vi "Default Text Formats.vi"(8 "Error In":errorcluster, 11 "Theme (Light)":string="Light Theme") -> (0 "Error Out":errorcluster, 1 "Base Themes":T1[](array[typedef]) {"[Named Text Styles]"."Text Formatting"."Font Size" min=6.0 step=1.0}, 3 "Notebook Theme":T1 {"[Named Text Styles]"."Text Formatting"."Font Size" min=6.0 step=1.0})   [LabVIEW 2021, in "Notebook.lvlib"]
uses:
  Notebook.lvlib
  Notebook Theme.ctl
  Rich Text Box/Named Text Style.ctl
  Rich Text Box/Text Formatting.ctl
  Rich Text Box/Text Colors.ctl
  Rich Text Box/Text Style.ctl
  Rich Text Box/Text Alignment.ctl
  Rich Text Box/Rich Text Box.lvlib
panel:
  # "see the License on the block diagram (Ctrl+E or Window:Show Block Diagram)"
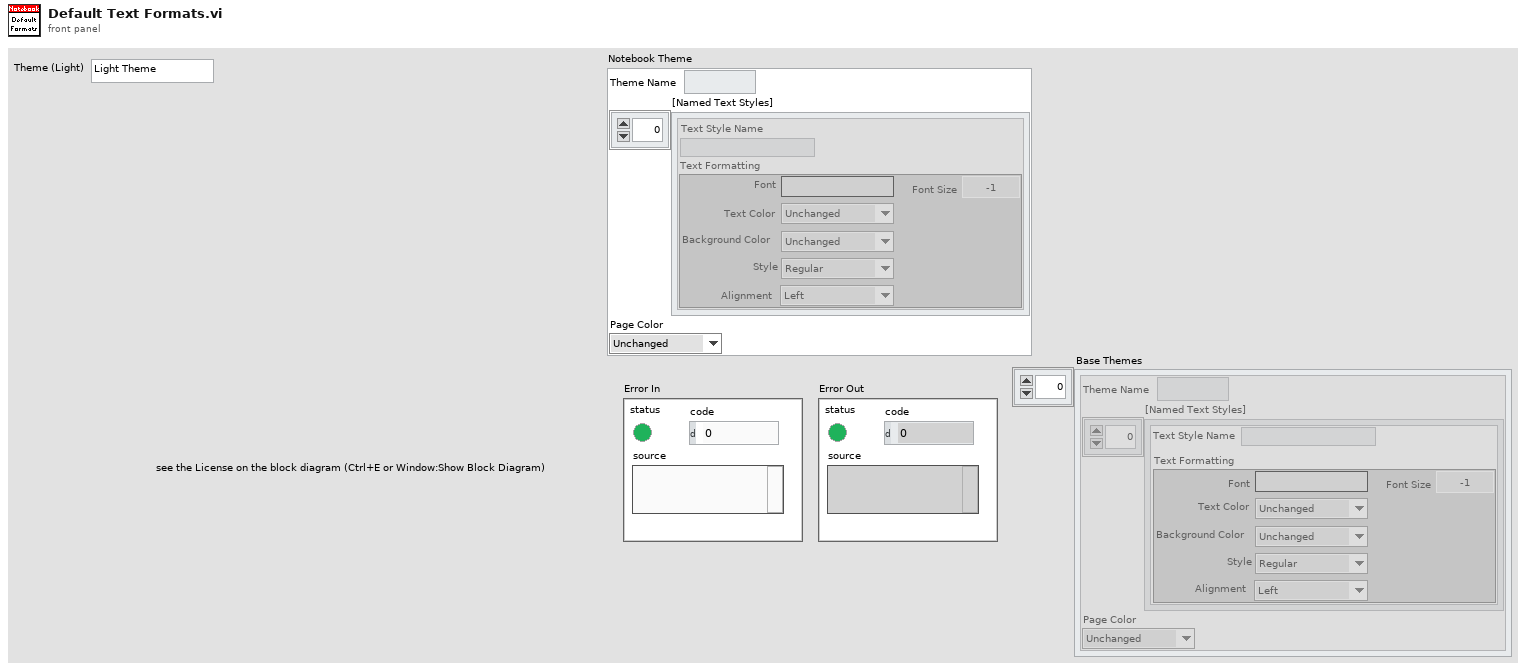
[diagram p1: front panel]
types:
  T1 = typedef "Notebook.lvlib/Notebook Theme.ctl" = cluster{"Theme Name":string, "[Named Text Styles]":T2[], "Page Color":T4}
  T2 = typedef "Notebook.lvlib/Named Text Style.ctl" = cluster{"Text Formatting":T3, "Text Style Name":string}
  T3 = typedef "Rich Text Box.lvlib/Text Formatting.ctl" = cluster{"Font":string, "Text Color":T4, "Background Color":T4, "Style":T5, "Font Size":dbl, "Alignment":T6}
  T4 = typedef "Rich Text Box.lvlib/Text Colors.ctl" = enum16{"Unchanged", "Black", "Blue", "Cyan", "Maroon", "Gray", "Violet", "Green", "Light Green", "Orange", "Yellow", "Magenta", "Red", "White"}
  T5 = typedef "Rich Text Box.lvlib/Text Style.ctl" = enum16{"Regular", "Bold", "Italic", "Underline", "Strikeout"}
  T6 = typedef "Rich Text Box.lvlib/Text Alignment.ctl" = enum16{"Left", "Right", "Center"}
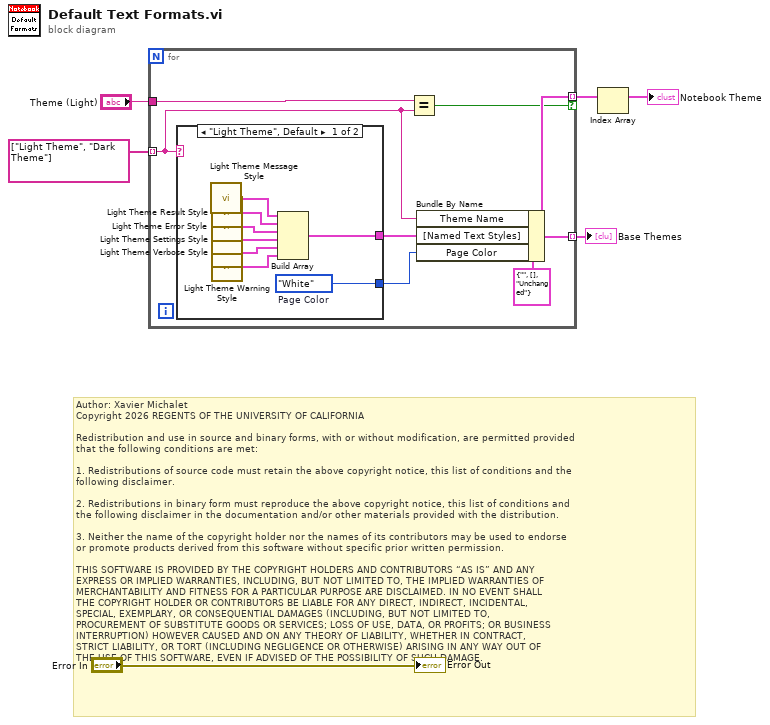
[diagram p0: block diagram]
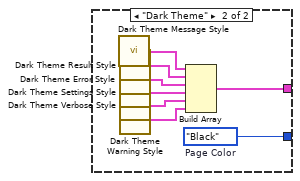
[diagram p2: hidden frame]
diagram:
  # "Author: Xavier Michalet\nCopyright 2026 REGENTS OF THE UNIVERSITY OF CALIFORNIA\n\nRedistribution and use in source and binary forms, with or without modification, are permitted provided\nthat the following conditions are met:\n\n1. Redistributions of source code must retain the above copyright notice, this list of conditions and the\nfollowing disclaimer.\n\n2. Redistributions in binary form must reproduce the above copyright notice, this list of conditions and\nthe following disclaimer in the documentation and/or other materials provided with the distribution.\n\n3. Neither the name of the copyright holder nor the names of its contributors may be used to endorse \nor promote products derived from this software without specific prior written permission.\n\nTHIS SOFTWARE IS PROVIDED BY THE COPYRIGHT HOLDERS AND CONTRIBUTORS “AS IS” AND ANY \nEXPRESS OR IMPLIED WARRANTIES, INCLUDING, BUT NOT LIMITED TO, THE IMPLIED WARRANTIES OF\nMERCHANTABILITY AND FITNESS FOR A PARTICULAR PURPOSE ARE DISCLAIMED. IN NO EVENT SHALL\nTHE COPYRIGHT HOLDER OR CONTRIBUTORS BE LIABLE FOR ANY DIRECT, INDIRECT, INCIDENTAL, \nSPECIAL, EXEMPLARY, OR CONSEQUENTIAL DAMAGES (INCLUDING, BUT NOT LIMITED TO, \nPROCUREMENT OF SUBSTITUTE GOODS OR SERVICES; LOSS OF USE, DATA, OR PROFITS; OR BUSINESS\nINTERRUPTION) HOWEVER CAUSED AND ON ANY THEORY OF LIABILITY, WHETHER IN CONTRACT, \nSTRICT LIABILITY, OR TORT (INCLUDING NEGLIGENCE OR OTHERWISE) ARISING IN ANY WAY OUT OF\nTHE USE OF THIS SOFTWARE, EVEN IF ADVISED OF THE POSSIBILITY OF SUCH DAMAGE."
  n1 = for {
    tunnel: string[] ["Light Theme", "Dark Theme"] ("Theme (Light)") -> [w10] mode=indexing
    tunnel: [w8] -> w4 mode=indexing
    tunnel: "Theme (Light)" -> [w9]
    tunnel: [w8] -> w2 mode=indexing if=w7
    n2 = case shown="\"Light Theme\", Default" w10 {
      tunnel: [w21 w29] -> w13
      tunnel: [w14 w22] -> w12
      frame "Light Theme", Default {
        w14 = Text_Colors."White"  # Page Color
        n3 = call "Light Theme Message Style.vi"() -> ("Text Style"=w15:T2)
        n4 = call "Light Theme Result Style.vi"() -> ("Text Style"=w16:T2)
        n5 = call "Light Theme Error Style.vi"() -> ("Text Style"=w17:T2)
        n6 = call "Light Theme Settings Style.vi"() -> ("Text Style"=w18:T2)
        n7 = call "Light Theme Verbose Style.vi"() -> ("Text Style"=w19:T2)
        n8 = call "Light Theme Warning Style.vi"() -> ("Text Style"=w20:T2)
        n9 = Build Array(w15, w16, w17, w18, w19, w20) -> (w21:T2[])
      }
      frame "Dark Theme" {
        w22 = Text_Colors."Black"  # Page Color
        n10 = call "Dark Theme Message Style.vi"() -> ("Text Style"=w23:T2)
        n11 = call "Dark Theme Result Style.vi"() -> ("Text Style"=w24:T2)
        n12 = call "Dark Theme Error Style.vi"() -> ("Text Style"=w25:T2)
        n13 = call "Dark Theme Settings Style.vi"() -> ("Text Style"=w26:T2)
        n14 = call "Dark Theme Verbose Style.vi"() -> ("Text Style"=w27:T2)
        n15 = call "Dark Theme Warning Style.vi"() -> ("Text Style"=w28:T2)
        n16 = Build Array(w23, w24, w25, w26, w27, w28) -> (w29:T2[])
      }
    }
    n17 = Equal?(x=w9, y=w10) -> (x = y?=w7:bool)
    n18 = Bundle By Name(cluster=T1 {"Theme Name"="", "[Named Text Styles]"=[], "Page Color"=enum."Unchanged"} ("Notebook Theme"), "Theme Name"=w10, "[Named Text Styles]"=w13, "Page Color"=w12) -> (w8:T1)
  }
  "Base Themes" <- w4
  n19 = Index Array(array=w2) -> (element=→"Notebook Theme":T1)  [unwired: 1 in]
  "Error Out" <- "Error In"
